vi "auto.vi"() -> ()   [LabVIEW 2010, in "LASA Beta.lvrbt"]
uses:
  LASA Beta.lvrbt
  <vilib>/NXT/Block Support/NXT_ButtonSelector.ctl
  <vilib>/NXT/Dual Mode Library/Display/clearDisplay.vi
  <vilib>/NXT/Dual Mode Library/Display/drawText.vi
  <vilib>/NXT/Dual Mode Library/Sensors/readNXTButton.vi
  <vilib>/NXT/Dual Mode Library/Waits/Wait_Num(msec).vi
  <vilib>/NXT/Dual Mode Library/Display/drawNumber.vi
  op-init.vi
  op-run.vi
  op-read.vi
panel:
  out "IR Success":bool
  in  "Distance":dbl=5750.0
  out "Enabled":bool
  out "Team Number":string="4290"
  in  "Other":dbl
  in  "Ramp":dbl
  in  "Direction":dbl
  in  "Time Delay":dbl
  in  "Cursor":dbl
  # "INITIALIZATION"
  # "Set this number to display team information"
  # "AUTONOMOUS"
  # "If enabled, use robot is on as read by comm. loop"
  # "Data from current IR sensor"
  # "Controller state as read by the comm. loop"
  # "Distance Needed to Travel from Start to B1\nEncoder Counts (1/4th degrees)"
  # "Turns ON when IR is detected"
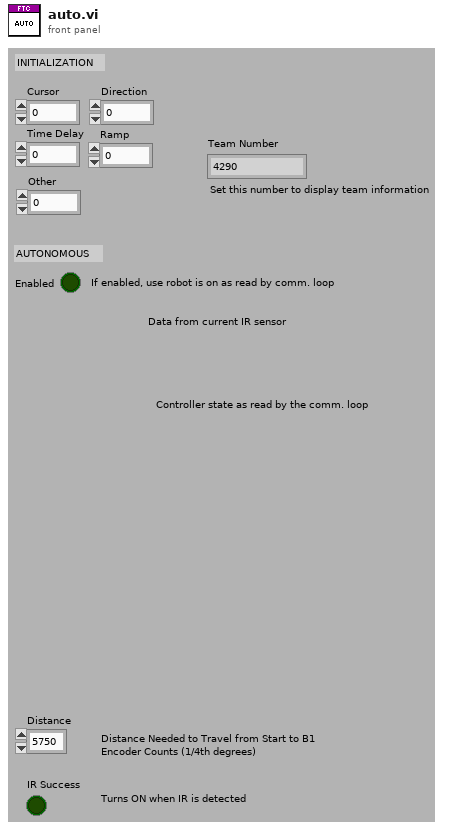
[diagram p1: front panel]
types:
  T1 = typedef "NXT_ButtonSelector.ctl" = u16
  T2 = typedef "LVHSConnector.ctl" = cluster{"Hardware":string, "Flattened String":string}
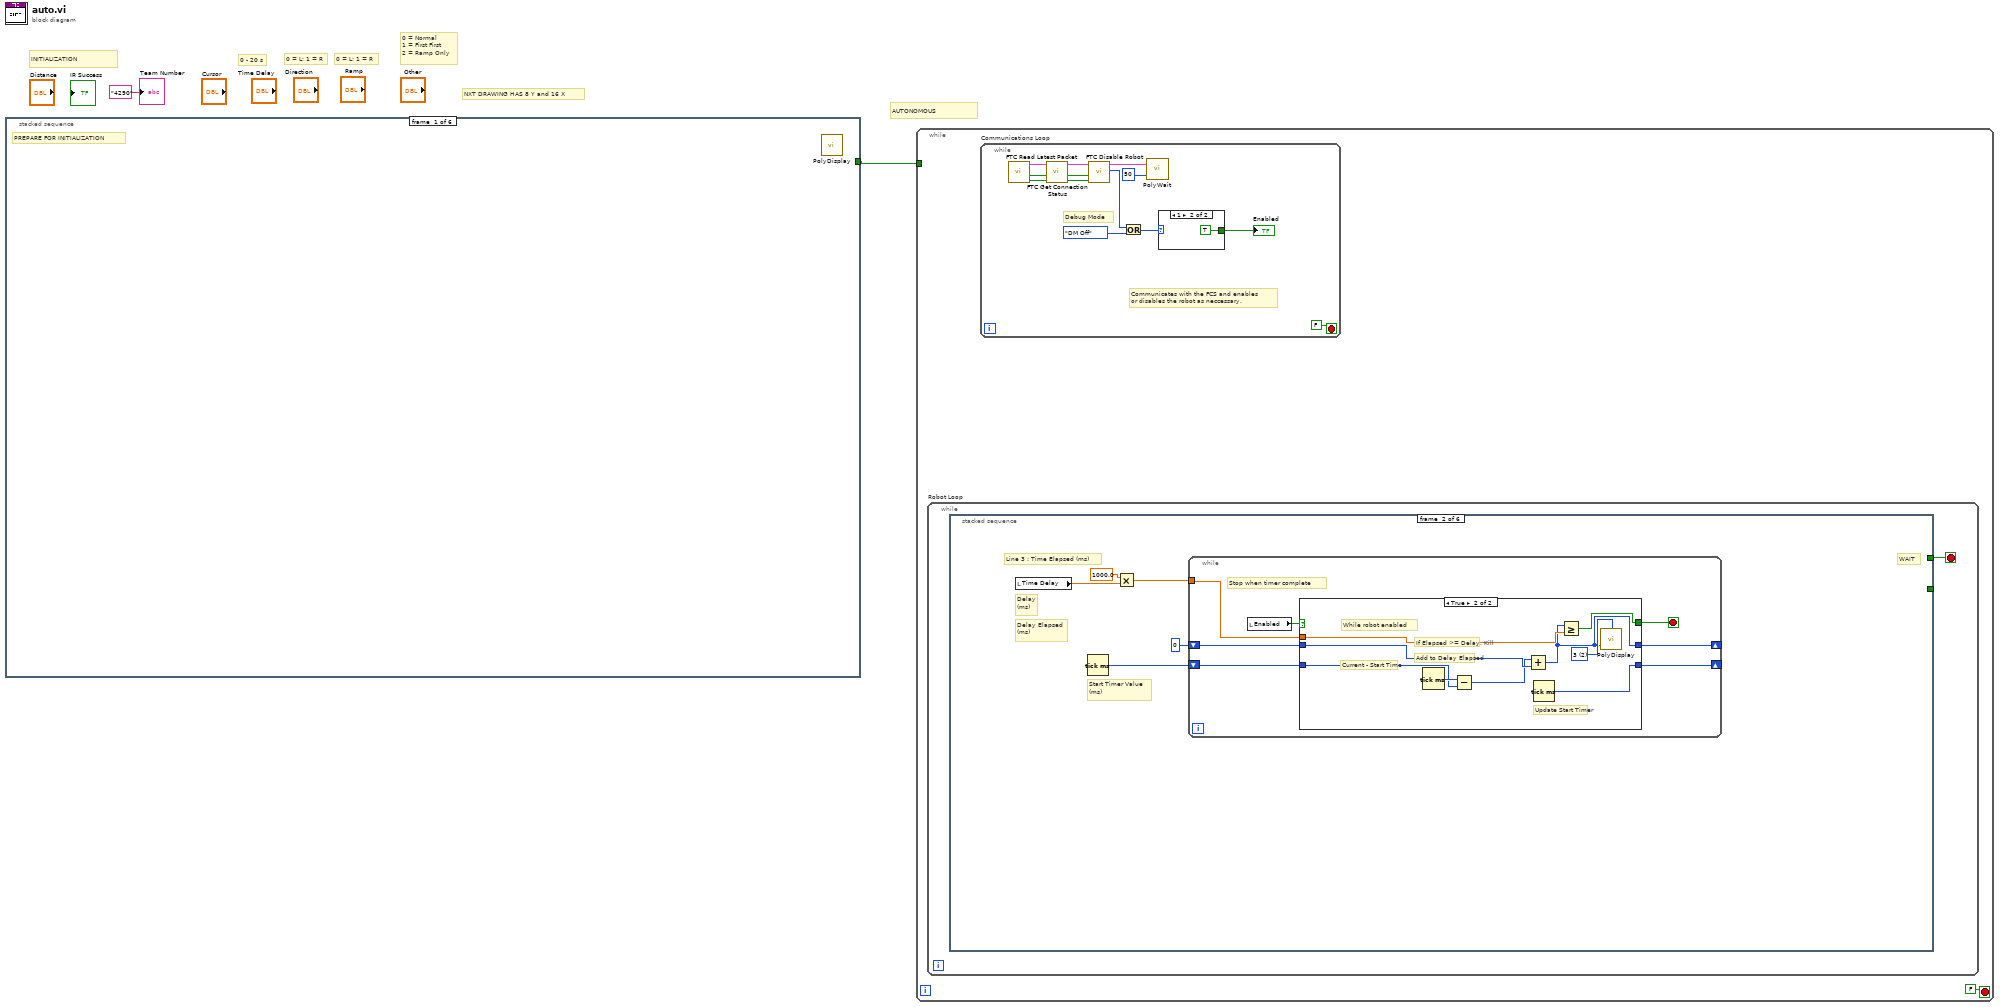
[diagram p0: block diagram]
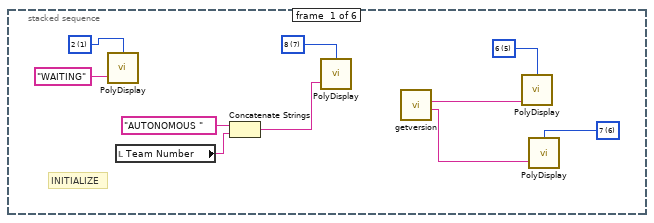
[diagram p2: hidden frame]
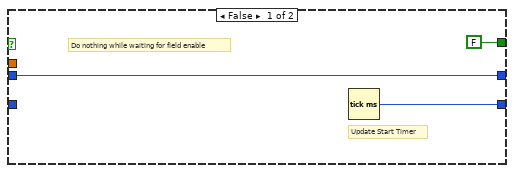
[diagram p3: hidden frame]
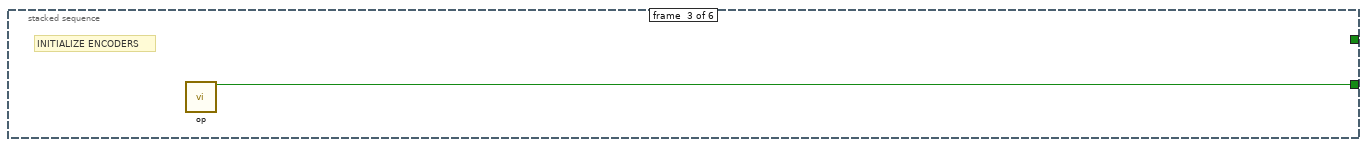
[diagram p4: hidden frame]
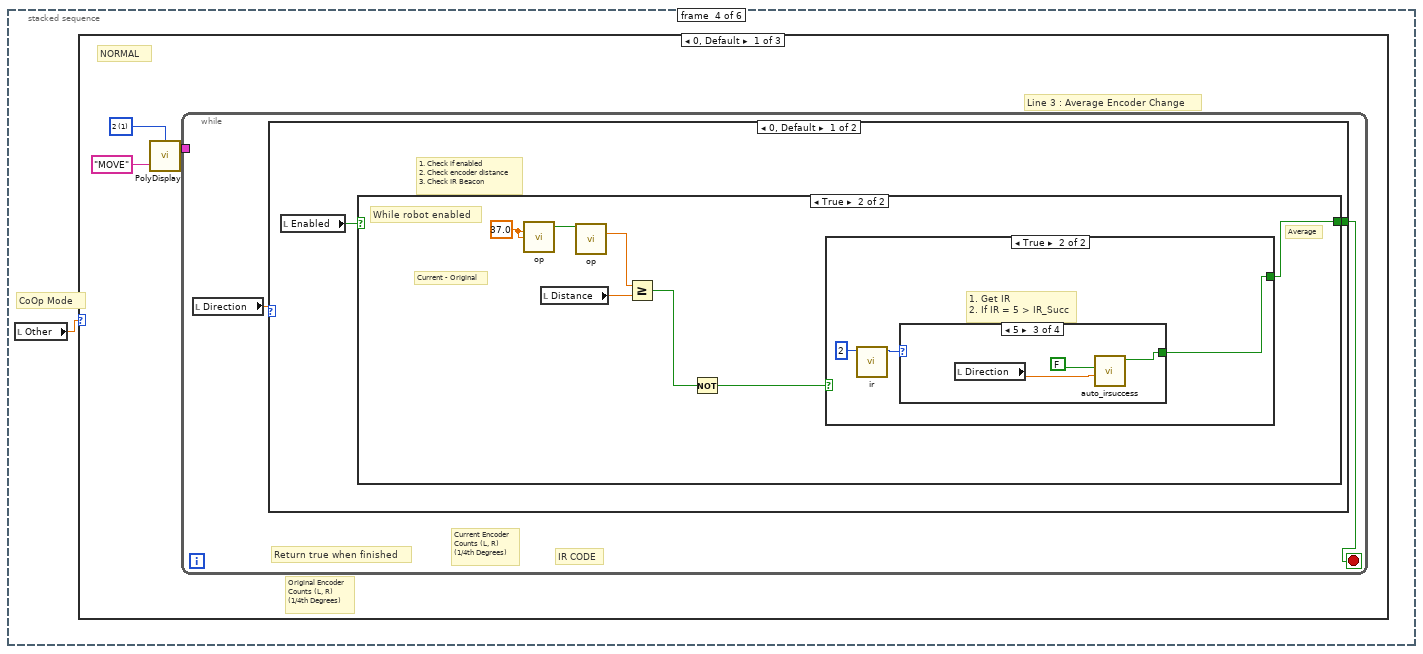
[diagram p5: hidden frame]
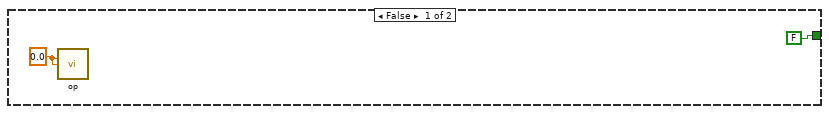
[diagram p6: hidden frame]
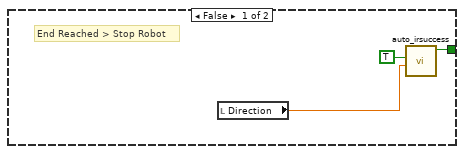
[diagram p7: hidden frame]
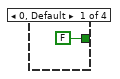
[diagram p8: hidden frame]
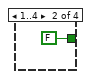
[diagram p9: hidden frame]
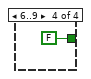
[diagram p10: hidden frame]
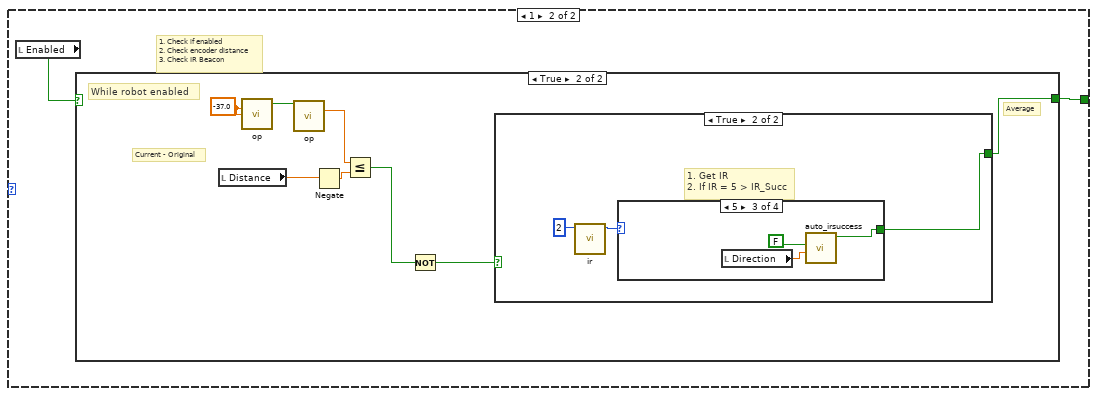
[diagram p11: hidden frame]
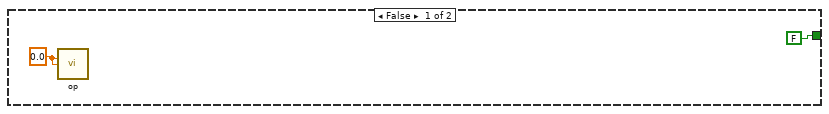
[diagram p12: hidden frame]
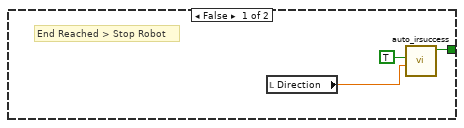
[diagram p13: hidden frame]
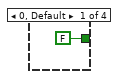
[diagram p14: hidden frame]
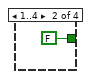
[diagram p15: hidden frame]
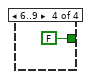
[diagram p16: hidden frame]
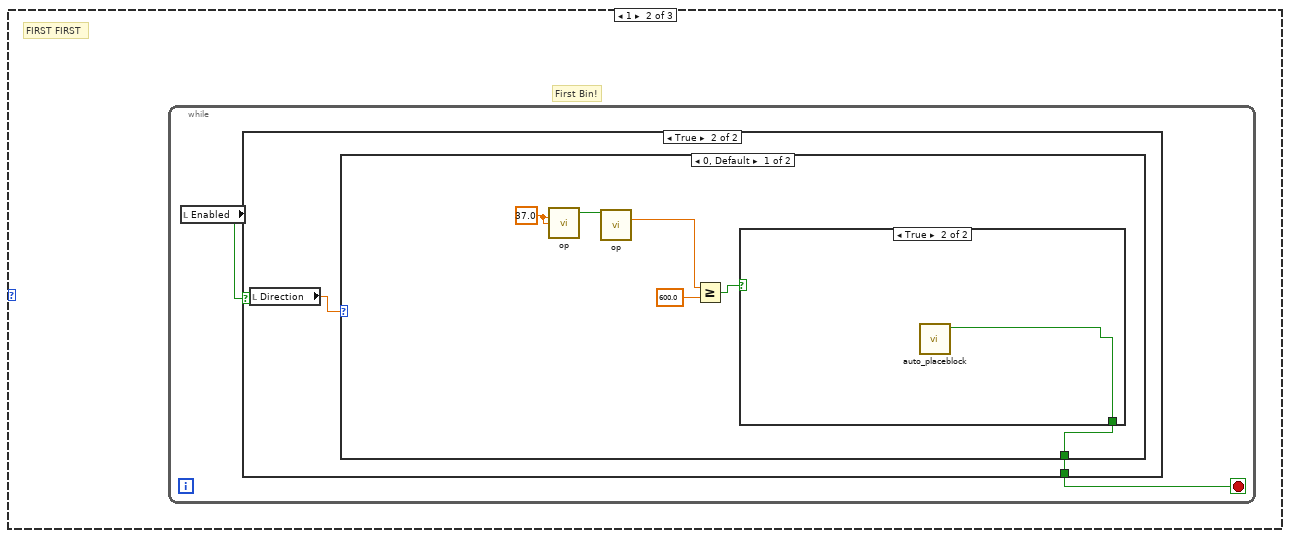
[diagram p17: hidden frame]
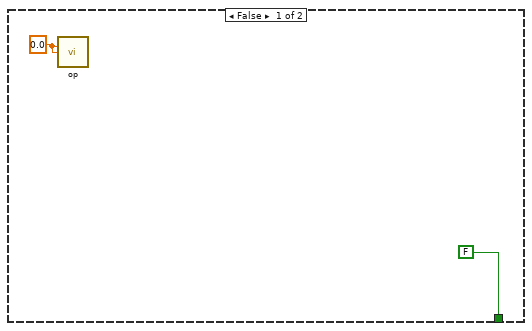
[diagram p18: hidden frame]
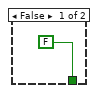
[diagram p19: hidden frame]
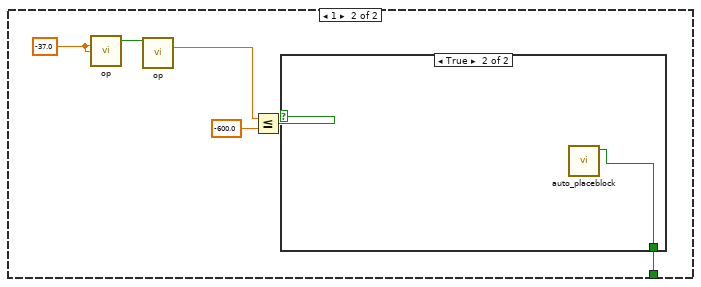
[diagram p20: hidden frame]
diagram:
  # "0 = Normal\n1 = First First\n2 = Ramp Only"
  # "AUTONOMOUS"
  # "INITIALIZATION"
  # "NXT DRAWING HAS 8 Y and 16 X"
  # "0 = L; 1 = R"
  # "0 - 20 s"
  # "0 = L; 1 = R"
  n1 = stacked-sequence {
    tunnel: [_ _ _ _ _ w144] -> w1
    frame #0 {
      # "PREPARE FOR INITIALIZATION"
      n2 = call-poly <vilib>:"PolyDisplay.vi"() -> ()  [unwired: 4 in, 1 out]
    }
    frame #1 {
      n3 = stacked-sequence {
        frame #0 {
          w3 = i16 7 items=["1", "2", "3", "4", "5", "6", "7", "8"] ("Line")
          w11 = i16 2 items=["1", "2", "3", "4", "5", "6", "7", "8"] ("Line")
          w9 = i16 0 items=["1", "2", "3", "4", "5", "6", "7", "8"] ("Line")
          # "-_0 sec_+"
          n4 = local write "Cursor"(0.0 ("Cursor")) -> ()
          n5 = call-poly <vilib>:"PolyDisplay.vi"("Text"="- 0 sec +", "Line"=w11) -> ()  [unwired: 2 in, 1 out]
          n6 = local read "Team Number"() -> (w5:string)
          n7 = call-poly <vilib>:"PolyDisplay.vi"("Text"="TIME DELAY", "Line"=w9) -> ()  [unwired: 2 in, 1 out]
          n8 = Concatenate Strings("AUTONOMOUS " ("string"), w5) -> (w6:string)
          n9 = call-poly <vilib>:"PolyDisplay.vi"("Text"=w6, "Line"=w3) -> ()  [unwired: 2 in, 1 out]
        }
        frame #1 {
          n10 = while {
            stop <- w16 stop-if-true
            w13 = T1 1 items=["Enter button"=3, "Left button"=2, "Right button"=1] ("Button (Enter button)")
            w15 = T1 2 items=["Enter button"=3, "Left button"=2, "Right button"=1] ("Button (Enter button)")
            w18 = T1 3 items=["Enter button"=3, "Left button"=2, "Right button"=1] ("Button (Enter button)")
            n11 = call-poly <vilib>:"PolySensor.vi"("Button (Enter button)"=w15) -> ("Yes/No"=w14:bool)  [unwired: 2 in, 1 out]
            n12 = call-poly <vilib>:"PolySensor.vi"("Button (Enter button)"=w13) -> ("Yes/No"=w12:bool)  [unwired: 2 in, 1 out]
            n13 = call-poly <vilib>:"PolySensor.vi"("Button (Enter button)"=w18) -> ("Yes/No"=w17:bool)  [unwired: 2 in, 1 out]
            n14 = case shown="True" w14 {
              frame False {
              }
              frame True {
                n15 = local read "Cursor"() -> (w41:dbl)
                n16 = Greater?(x=w41, y=0.0) -> (0:w40:bool)
                n17 = case shown="True" w40 {
                  frame False {
                  }
                  frame True {
                    w45 = i16 2 items=["1", "2", "3", "4", "5", "6", "7", "8"] ("Line")
                    n18 = local read "Cursor"() -> (w50:dbl)
                    n19 = Wait (ms)(milliseconds to wait=u32 300) -> ()  [unwired: 1 out]
                    n20 = Subtract(x=w50, y=5.0) -> (x-y=w49:dbl)
                    n21 = local write "Cursor"(w49) -> ()
                    n22 = call <vilib>:"NXT_floatToString.vi"("number"=w49) -> ("string"=w46:string)
                    n23 = Concatenate Strings("- " ("string"), w46, " sec +" ("string")) -> (w44:string)
                    n24 = call-poly <vilib>:"PolyDisplay.vi"("Text"=w44, "Line"=w45) -> ()  [unwired: 2 in, 1 out]
                  }
                }
              }
            }
            n25 = case shown="True" w12 {
              frame False {
              }
              frame True {
                n26 = local read "Cursor"() -> (w21:dbl)
                n27 = Less?(x=w21, y=20.0) -> (x < y?=w19:bool)
                n28 = case shown="True" w19 {
                  frame False {
                  }
                  frame True {
                    w25 = i16 2 items=["1", "2", "3", "4", "5", "6", "7", "8"] ("Line")
                    n29 = local read "Cursor"() -> (w29:dbl)
                    n30 = Wait (ms)(milliseconds to wait=u32 300) -> ()  [unwired: 1 out]
                    n31 = Add(x=w29, y=5.0) -> (x+y=w23:dbl)
                    n32 = local write "Cursor"(w23) -> ()
                    n33 = call <vilib>:"NXT_floatToString.vi"("number"=w23) -> ("string"=w27:string)
                    n34 = Concatenate Strings("- " ("string"), w27, " sec +" ("string")) -> (w26:string)
                    n35 = call-poly <vilib>:"PolyDisplay.vi"("Text"=w26, "Line"=w25) -> ()  [unwired: 2 in, 1 out]
                  }
                }
              }
            }
            n36 = case shown="True" w17 {
              tunnel: [FALSE w32] -> w16
              frame False {
              }
              frame True {
                n37 = stacked-sequence {
                  tunnel: [_ _ TRUE] -> w32
                  frame #0 {
                    n38 = local read "Cursor"() -> (w34:dbl)
                    n39 = local write "Direction"(0.0 ("Direction")) -> ()
                    n40 = local write "Time Delay"(w34) -> ()
                    n41 = call-poly <vilib>:"PolyDisplay.vi"() -> ()  [unwired: 4 in, 1 out]
                  }
                  frame #1 {
                    w37 = i16 0 items=["1", "2", "3", "4", "5", "6", "7", "8"] ("Line")
                    n42 = local write "Cursor"(0.0 ("Cursor")) -> ()
                    n43 = call-poly <vilib>:"PolyDisplay.vi"("Text"="Working...", "Line"=w37) -> ()  [unwired: 2 in, 1 out]
                  }
                  frame #2 {
                    n44 = Wait (ms)(milliseconds to wait=u32 500) -> ()  [unwired: 1 out]
                  }
                }
              }
            }
          }
        }
      }
    }
    frame #2 {
      # "2 = L/R"
      n45 = stacked-sequence {
        frame #0 {
          w52 = i16 3 items=["1", "2", "3", "4", "5", "6", "7", "8"] ("Line")
          w57 = i16 7 items=["1", "2", "3", "4", "5", "6", "7", "8"] ("Line")
          w61 = i16 2 items=["1", "2", "3", "4", "5", "6", "7", "8"] ("Line")
          w59 = i16 0 items=["1", "2", "3", "4", "5", "6", "7", "8"] ("Line")
          n46 = local read "Team Number"() -> (w54:string)
          n47 = call-poly <vilib>:"PolyDisplay.vi"("Text"="[LEFT] = L", "Line"=w61) -> ()  [unwired: 2 in, 1 out]
          n48 = call-poly <vilib>:"PolyDisplay.vi"("Text"="[RIGHT] = R", "Line"=w52) -> ()  [unwired: 2 in, 1 out]
          n49 = Concatenate Strings("AUTONOMOUS " ("string"), w54) -> (w53:string)
          n50 = call-poly <vilib>:"PolyDisplay.vi"("Text"="START LOCATION", "Line"=w59) -> ()  [unwired: 2 in, 1 out]
          n51 = call-poly <vilib>:"PolyDisplay.vi"("Text"=w53, "Line"=w57) -> ()  [unwired: 2 in, 1 out]
        }
        frame #1 {
          n52 = while {
            stop <- w62 stop-if-true
            w67 = T1 1 items=["Enter button"=3, "Left button"=2, "Right button"=1] ("Button (Enter button)")
            w68 = T1 2 items=["Enter button"=3, "Left button"=2, "Right button"=1] ("Button (Enter button)")
            n53 = call-poly <vilib>:"PolySensor.vi"("Button (Enter button)"=w68) -> ("Yes/No"=w65:bool)  [unwired: 2 in, 1 out]
            n54 = call-poly <vilib>:"PolySensor.vi"("Button (Enter button)"=w67) -> ("Yes/No"=w66:bool)  [unwired: 2 in, 1 out]
            n55 = case shown="True" w65 {
              tunnel: [FALSE TRUE] -> w64
              frame False {
              }
              frame True {
                n56 = local write "Direction"(0.0 ("Direction")) -> ()
              }
            }
            n57 = case shown="True" w66 {
              tunnel: [FALSE TRUE] -> w63
              frame False {
              }
              frame True {
                n58 = local write "Direction"(1.0 ("Direction")) -> ()
              }
            }
            n59 = Or(x=w64, y=w63) -> (x .or. y?=w62:bool)
          }
        }
        frame #2 {
          n60 = local write "Cursor"(0.0 ("Cursor")) -> ()
          n61 = local write "Ramp"(0.0 ("Ramp")) -> ()
          n62 = call-poly <vilib>:"PolyDisplay.vi"() -> ()  [unwired: 4 in, 1 out]
        }
        frame #3 {
          w78 = i16 0 items=["1", "2", "3", "4", "5", "6", "7", "8"] ("Line")
          n63 = call-poly <vilib>:"PolyDisplay.vi"("Text"="Working...", "Line"=w78) -> ()  [unwired: 2 in, 1 out]
        }
        frame #4 {
          n64 = Wait (ms)(milliseconds to wait=u32 500) -> ()  [unwired: 1 out]
        }
      }
    }
    frame #3 {
      # "3 = Force On Ramp (L/R)"
      n65 = stacked-sequence {
        frame #0 {
          w81 = i16 3 items=["1", "2", "3", "4", "5", "6", "7", "8"] ("Line")
          w85 = i16 7 items=["1", "2", "3", "4", "5", "6", "7", "8"] ("Line")
          w89 = i16 2 items=["1", "2", "3", "4", "5", "6", "7", "8"] ("Line")
          w87 = i16 0 items=["1", "2", "3", "4", "5", "6", "7", "8"] ("Line")
          n66 = local read "Team Number"() -> (w80:string)
          n67 = call-poly <vilib>:"PolyDisplay.vi"("Text"="[RIGHT] = R", "Line"=w81) -> ()  [unwired: 2 in, 1 out]
          n68 = call-poly <vilib>:"PolyDisplay.vi"("Text"="FORCE RAMP", "Line"=w87) -> ()  [unwired: 2 in, 1 out]
          n69 = call-poly <vilib>:"PolyDisplay.vi"("Text"="[LEFT] = L", "Line"=w89) -> ()  [unwired: 2 in, 1 out]
          n70 = Concatenate Strings("AUTONOMOUS " ("string"), w80) -> (w82:string)
          n71 = call-poly <vilib>:"PolyDisplay.vi"("Text"=w82, "Line"=w85) -> ()  [unwired: 2 in, 1 out]
        }
        frame #1 {
          n72 = while {
            stop <- w90 stop-if-true
            w95 = T1 1 items=["Enter button"=3, "Left button"=2, "Right button"=1] ("Button (Enter button)")
            w96 = T1 2 items=["Enter button"=3, "Left button"=2, "Right button"=1] ("Button (Enter button)")
            n73 = call-poly <vilib>:"PolySensor.vi"("Button (Enter button)"=w96) -> ("Yes/No"=w94:bool)  [unwired: 2 in, 1 out]
            n74 = call-poly <vilib>:"PolySensor.vi"("Button (Enter button)"=w95) -> ("Yes/No"=w93:bool)  [unwired: 2 in, 1 out]
            n75 = case shown="True" w94 {
              tunnel: [FALSE TRUE] -> w92
              frame False {
              }
              frame True {
                n76 = local write "Ramp"(0.0 ("Ramp")) -> ()
              }
            }
            n77 = case shown="True" w93 {
              tunnel: [FALSE TRUE] -> w91
              frame False {
              }
              frame True {
                n78 = local write "Ramp"(1.0 ("Ramp")) -> ()
              }
            }
            n79 = Or(x=w92, y=w91) -> (x .or. y?=w90:bool)
          }
        }
        frame #2 {
          n80 = local write "Cursor"(0.0 ("Cursor")) -> ()
          n81 = local write "Other"(0.0 ("Other")) -> ()
          n82 = call-poly <vilib>:"PolyDisplay.vi"() -> ()  [unwired: 4 in, 1 out]
        }
        frame #3 {
          w106 = i16 0 items=["1", "2", "3", "4", "5", "6", "7", "8"] ("Line")
          n83 = call-poly <vilib>:"PolyDisplay.vi"("Text"="Working...", "Line"=w106) -> ()  [unwired: 2 in, 1 out]
        }
        frame #4 {
          n84 = Wait (ms)(milliseconds to wait=u32 500) -> ()  [unwired: 1 out]
        }
      }
    }
    frame #4 {
      # "4 = Ramp Only, First Bin, or Normal"
      n85 = stacked-sequence {
        frame #0 {
          w108 = i16 4 items=["1", "2", "3", "4", "5", "6", "7", "8"] ("Line")
          w111 = i16 3 items=["1", "2", "3", "4", "5", "6", "7", "8"] ("Line")
          w115 = i16 7 items=["1", "2", "3", "4", "5", "6", "7", "8"] ("Line")
          w119 = i16 2 items=["1", "2", "3", "4", "5", "6", "7", "8"] ("Line")
          w117 = i16 0 items=["1", "2", "3", "4", "5", "6", "7", "8"] ("Line")
          n86 = local read "Team Number"() -> (w110:string)
          n87 = call-poly <vilib>:"PolyDisplay.vi"("Text"="[L] = First Bin", "Line"=w111) -> ()  [unwired: 2 in, 1 out]
          n88 = Concatenate Strings("AUTONOMOUS " ("string"), w110) -> (w112:string)
          n89 = call-poly <vilib>:"PolyDisplay.vi"("Text"="[R] = Ramp Only", "Line"=w108) -> ()  [unwired: 2 in, 1 out]
          n90 = call-poly <vilib>:"PolyDisplay.vi"("Text"="COOPERATION MODE", "Line"=w117) -> ()  [unwired: 2 in, 1 out]
          n91 = call-poly <vilib>:"PolyDisplay.vi"("Text"="[ENTER] = Normal", "Line"=w119) -> ()  [unwired: 2 in, 1 out]
          n92 = call-poly <vilib>:"PolyDisplay.vi"("Text"=w112, "Line"=w115) -> ()  [unwired: 2 in, 1 out]
        }
        frame #1 {
          n93 = while {
            stop <- w124 stop-if-true
            w128 = T1 3 items=["Enter button"=3, "Left button"=2, "Right button"=1] ("Button (Enter button)")
            w129 = T1 1 items=["Enter button"=3, "Left button"=2, "Right button"=1] ("Button (Enter button)")
            w130 = T1 2 items=["Enter button"=3, "Left button"=2, "Right button"=1] ("Button (Enter button)")
            n94 = call-poly <vilib>:"PolySensor.vi"("Button (Enter button)"=w130) -> ("Yes/No"=w127:bool)  [unwired: 2 in, 1 out]
            n95 = call-poly <vilib>:"PolySensor.vi"("Button (Enter button)"=w129) -> ("Yes/No"=w126:bool)  [unwired: 2 in, 1 out]
            n96 = case shown="True" w127 {
              tunnel: [FALSE TRUE] -> w121
              frame False {
              }
              frame True {
                n97 = local write "Other"(1.0 ("Other")) -> ()
              }
            }
            n98 = case shown="True" w126 {
              tunnel: [FALSE TRUE] -> w120
              frame False {
              }
              frame True {
                n99 = local write "Other"(2.0 ("Other")) -> ()
              }
            }
            n100 = call-poly <vilib>:"PolySensor.vi"("Button (Enter button)"=w128) -> ("Yes/No"=w125:bool)  [unwired: 2 in, 1 out]
            n101 = case shown="True" w125 {
              tunnel: [FALSE TRUE] -> w122
              frame False {
              }
              frame True {
                n102 = local write "Other"(0.0 ("Other")) -> ()
              }
            }
            n103 = Or(x=w121, y=w120) -> (x .or. y?=w123:bool)
            n104 = Or(x=w123, y=w122) -> (x .or. y?=w124:bool)
          }
        }
        frame #2 {
          n105 = local write "Cursor"(0.0 ("Cursor")) -> ()
          n106 = call-poly <vilib>:"PolyDisplay.vi"() -> ()  [unwired: 4 in, 1 out]
        }
        frame #3 {
          w142 = i16 0 items=["1", "2", "3", "4", "5", "6", "7", "8"] ("Line")
          n107 = call-poly <vilib>:"PolyDisplay.vi"("Text"="Working...", "Line"=w142) -> ()  [unwired: 2 in, 1 out]
        }
        frame #4 {
          n108 = Wait (ms)(milliseconds to wait=u32 500) -> ()  [unwired: 1 out]
        }
      }
    }
    frame #5 {
      # "ENTER AUTONOMOUS"
      n109 = stacked-sequence {
        tunnel: [_ _ FALSE] -> w144
        frame #0 {
          n110 = call-poly <vilib>:"PolyDisplay.vi"() -> ()  [unwired: 4 in, 1 out]
        }
        frame #1 {
          w148 = i16 7 items=["1", "2", "3", "4", "5", "6", "7", "8"] ("Line")
          n111 = local read "Team Number"() -> (w145:string)
          n112 = Concatenate Strings("AUTONOMOUS " ("string"), w145) -> (w146:string)
          n113 = call-poly <vilib>:"PolyDisplay.vi"("Text"=w146, "Line"=w148) -> ()  [unwired: 2 in, 1 out]
        }
        frame #2 {
        }
      }
    }
  }
  n114 = while {
    tunnel: w1 -> [_]
    stop <- FALSE stop-if-true
    n115 = while "Robot Loop" {
      stop <- w151 stop-if-true
      n116 = stacked-sequence {
        tunnel: [_ _ _ _ _ TRUE] -> w151
        tunnel: [_ _ w186 _ _ _] -> _
        frame #0 {
          w152 = i16 5 items=["1", "2", "3", "4", "5", "6", "7", "8"] ("Line")
          w153 = i16 6 items=["1", "2", "3", "4", "5", "6", "7", "8"] ("Line")
          w159 = i16 7 items=["1", "2", "3", "4", "5", "6", "7", "8"] ("Line")
          w161 = i16 1 items=["1", "2", "3", "4", "5", "6", "7", "8"] ("Line")
          # "INITIALIZE"
          n117 = call-poly <vilib>:"PolyDisplay.vi"("Text"="WAITING", "Line"=w161) -> ()  [unwired: 2 in, 1 out]
          n118 = local read "Team Number"() -> (w157:string)
          n119 = Concatenate Strings("AUTONOMOUS " ("string"), w157) -> (w156:string)
          n120 = call-poly <vilib>:"PolyDisplay.vi"("Text"=w156, "Line"=w159) -> ()  [unwired: 2 in, 1 out]
          n121 = call "getversion.vi"() -> ("Revision"=w154:string, "Version"=w155:string)  [unwired: 9 in, 1 out]
          n122 = call-poly <vilib>:"PolyDisplay.vi"("Text"=w155, "Line"=w152) -> ()  [unwired: 2 in, 1 out]
          n123 = call-poly <vilib>:"PolyDisplay.vi"("Text"=w154, "Line"=w153) -> ()  [unwired: 2 in, 1 out]
        }
        frame #1 {
          # "Line 3 : Time Elapsed (ms)"
          # "Delay\n(ms)"
          # "Start Timer Value\n(ms)"
          # "Delay Elapsed\n(ms)"
          # "WAIT"
          n124 = local read "Time Delay"() -> (w165:dbl)
          n125 = Tick Count (ms)() -> (millisecond timer value=w162:u32)
          n126 = Multiply(x=1000.0, y=w165) -> (x*y=w163:dbl)
          n127 = while {
            shift-right: [w167] -> _
            shift-left: 0 -> [w170]
            tunnel: w163 -> [w172]
            shift-right: [w169] -> _
            shift-left: w162 -> [w171]
            stop <- w168 stop-if-true
            # "Stop when timer complete"
            n128 = local read "Enabled"() -> (w173:bool)
            n129 = case shown="True" w173 {
              tunnel: w172 -> [_ w181]
              tunnel: w171 -> [_ w182]
              tunnel: w170 -> [w175 w184]
              tunnel: [w176 w179] -> w169
              tunnel: [FALSE w180] -> w168
              tunnel: [w175 w177] -> w167
              frame False {
                # "Do nothing while waiting for field enable"
                # "Update Start Timer"
                n130 = Tick Count (ms)() -> (millisecond timer value=w176:u32)
              }
              frame True {
                w178 = i16 2 items=["1", "2", "3", "4", "5", "6", "7", "8"] ("Line")
                # "Update Start Timer"
                # "If Elapsed >= Delay, Kill"
                # "Add to Delay Elapsed"
                # "Current - Start Time"
                # "While robot enabled"
                n131 = Tick Count (ms)() -> (millisecond timer value=w185:u32)
                n132 = Subtract(x=w185, y=w182) -> (x-y=w183:u32)
                n133 = Add(x=w183, y=w184) -> (x+y=w177:u32)
                n134 = Tick Count (ms)() -> (millisecond timer value=w179:u32)
                n135 = Greater Or Equal?(x=w177, y=w181) -> (x >= y?=w180:bool)
                n136 = call-poly <vilib>:"PolyDisplay.vi"("number"=w177, "Line"=w178) -> ()  [unwired: 2 in, 1 out]
              }
            }
          }
        }
        frame #2 {
          # "INITIALIZE ENCODERS"
          n137 = call-poly "op.vi"() -> ("Chain OUT"=w186:bool)  [unwired: 15 in]
        }
        frame #3 {
          # "CoOp Mode"
          n138 = local read "Other"() -> (w187:dbl)
          n139 = case shown="0, Default" w187 {
            frame 0, Default {
              w190 = i16 1 items=["1", "2", "3", "4", "5", "6", "7", "8"] ("Line")
              # "NORMAL"
              # "Line 3 : Average Encoder Change"
              # "Original Encoder\nCounts (L, R)\n(1/4th Degrees)"
              n140 = call-poly <vilib>:"PolyDisplay.vi"("Text"="MOVE", "Line"=w190) -> ("NXT"=w188:T2)  [unwired: 2 in]
              n141 = while {
                tunnel: w188 -> [_]
                stop <- w192 stop-if-true
                # "IR CODE"
                # "Current Encoder\nCounts (L, R)\n(1/4th Degrees)"
                # "Return true when finished"
                n142 = local read "Direction"() -> (w191:dbl)
                n143 = case shown="0, Default" w191 {
                  tunnel: [w193 w216] -> w192
                  frame 0, Default {
                    # "1. Check if enabled\n2. Check encoder distance\n3. Check IR Beacon"
                    n144 = local read "Enabled"() -> (w194:bool)
                    n145 = case shown="True" w194 {
                      tunnel: [FALSE w199] -> w193
                      frame False {
                        w195 = 0.0 ("Left Drive")
                        n146 = call-poly "op.vi"("Left Drive"=w195, "Right Drive"=w195) -> ()  [unwired: 13 in, 1 out]
                      }
                      frame True {
                        w203 = 37.0
                        # "Average"
                        # "Current - Original"
                        # "While robot enabled"
                        n147 = call-poly "op.vi"("Left Drive"=w203, "Right Drive"=w203) -> ("Chain OUT"=w198:bool)  [unwired: 13 in]
                        n148 = local read "Distance"() -> (w202:dbl)
                        n149 = call-poly "op.vi"("Chain IN"=w198) -> ("Encoder Left Drive"=w197:dbl)  [unwired: 8 in, 6 out]
                        n150 = Greater Or Equal?(x=w197, y=w202) -> (x >= y?=w201:bool)
                        n151 = Not(x=w201) -> (.not. x?=w200:bool)
                        n152 = case shown="True" w200 {
                          tunnel: [w205 w209] -> w199
                          frame False {
                            # "End Reached > Stop Robot"
                            n153 = local read "Direction"() -> (w204:dbl)
                            n154 = call "auto_irsuccess.vi"("Direction"=w204, "Skip IR"=TRUE) -> ("Success"=w205:bool)  [unwired: 9 in]
                          }
                          frame True {
                            # "1. Get IR\n2. If IR = 5 > IR_Succ"
                            n155 = call "ir.vi"("Port"=u8 2) -> ("Direction"=w208:i16)  [unwired: 10 in]
                            n156 = case shown="5" w208 {
                              tunnel: [FALSE ("Success") FALSE w214 FALSE] -> w209
                              frame 0, Default {
                              }
                              frame 1..4 {
                              }
                              frame 5 {
                                n157 = local read "Direction"() -> (w212:dbl)
                                n158 = call "auto_irsuccess.vi"("Direction"=w212, "Skip IR"=FALSE) -> ("Success"=w214:bool)  [unwired: 9 in]
                              }
                              frame 6..9 {
                              }
                            }
                          }
                        }
                      }
                    }
                  }
                  frame 1 {
                    # "1. Check if enabled\n2. Check encoder distance\n3. Check IR Beacon"
                    n159 = local read "Enabled"() -> (w217:bool)
                    n160 = case shown="True" w217 {
                      tunnel: [FALSE w223] -> w216
                      frame False {
                        w218 = 0.0 ("Left Drive")
                        n161 = call-poly "op.vi"("Left Drive"=w218, "Right Drive"=w218) -> ()  [unwired: 13 in, 1 out]
                      }
                      frame True {
                        w227 = -37.0
                        # "Average"
                        # "Current - Original"
                        # "While robot enabled"
                        n162 = local read "Distance"() -> (w226:dbl)
                        n163 = call-poly "op.vi"("Left Drive"=w227, "Right Drive"=w227) -> ("Chain OUT"=w222:bool)  [unwired: 13 in]
                        n164 = call-poly "op.vi"("Chain IN"=w222) -> ("Encoder Left Drive"=w221:dbl)  [unwired: 8 in, 6 out]
                        n165 = Negate(x=w226) -> (-x=w220:dbl)
                        n166 = Less Or Equal?(x=w221, y=w220) -> (x <= y?=w225:bool)
                        n167 = Not(x=w225) -> (.not. x?=w224:bool)
                        n168 = case shown="True" w224 {
                          tunnel: [w229 w233] -> w223
                          frame False {
                            # "End Reached > Stop Robot"
                            n169 = local read "Direction"() -> (w228:dbl)
                            n170 = call "auto_irsuccess.vi"("Direction"=w228, "Skip IR"=TRUE) -> ("Success"=w229:bool)  [unwired: 9 in]
                          }
                          frame True {
                            # "1. Get IR\n2. If IR = 5 > IR_Succ"
                            n171 = call "ir.vi"("Port"=u8 2) -> ("Direction"=w232:i16)  [unwired: 10 in]
                            n172 = case shown="5" w232 {
                              tunnel: [FALSE ("Success") FALSE w238 FALSE] -> w233
                              frame 0, Default {
                              }
                              frame 1..4 {
                              }
                              frame 5 {
                                n173 = local read "Direction"() -> (w236:dbl)
                                n174 = call "auto_irsuccess.vi"("Direction"=w236, "Skip IR"=FALSE) -> ("Success"=w238:bool)  [unwired: 9 in]
                              }
                              frame 6..9 {
                              }
                            }
                          }
                        }
                      }
                    }
                  }
                }
              }
            }
            frame 1 {
              # "FIRST FIRST"
              # "First Bin!"
              n175 = while {
                stop <- w241 stop-if-true
                n176 = local read "Enabled"() -> (w240:bool)
                n177 = case shown="True" w240 {
                  tunnel: [FALSE w244] -> w241
                  frame False {
                    w243 = 0.0 ("Left Drive")
                    n178 = call-poly "op.vi"("Left Drive"=w243, "Right Drive"=w243) -> ()  [unwired: 13 in, 1 out]
                  }
                  frame True {
                    n179 = local read "Direction"() -> (w245:dbl)
                    n180 = case shown="0, Default" w245 {
                      tunnel: [w246 w254] -> w244
                      frame 0, Default {
                        w251 = 37.0
                        n181 = call-poly "op.vi"("Left Drive"=w251, "Right Drive"=w251) -> ("Chain OUT"=w250:bool)  [unwired: 13 in]
                        n182 = call-poly "op.vi"("Chain IN"=w250) -> ("Encoder Left Drive"=w247:dbl)  [unwired: 8 in, 6 out]
                        n183 = Greater Or Equal?(x=w247, y=600.0) -> (x >= y?=w248:bool)
                        n184 = case shown="True" w248 {
                          tunnel: [FALSE w253] -> w246
                          frame False {
                          }
                          frame True {
                            n185 = call "auto_placeblock.vi"() -> ("Chain OUT"=w253:bool)  [unwired: 11 in]
                          }
                        }
                      }
                      frame 1 {
                        w259 = -37.0
                        n186 = call-poly "op.vi"("Left Drive"=w259, "Right Drive"=w259) -> ("Chain OUT"=w258:bool)  [unwired: 13 in]
                        n187 = call-poly "op.vi"("Chain IN"=w258) -> ("Encoder Left Drive"=w257:dbl)  [unwired: 8 in, 6 out]
                        n188 = Less Or Equal?(x=w257, y=-600.0) -> (x <= y?=w255:bool)
                        n189 = case shown="True" w255 {
                          tunnel: [FALSE w261] -> w254
                          frame False {
                          }
                          frame True {
                            n190 = call "auto_placeblock.vi"() -> ("Chain OUT"=w261:bool)  [unwired: 11 in]
                          }
                        }
                      }
                    }
                  }
                }
              }
            }
            frame 2 {
              # "Ramp Only, Skip"
            }
          }
        }
        frame #4 {
          w264 = i16 1 items=["1", "2", "3", "4", "5", "6", "7", "8"] ("Line")
          # "RAMP CODE"
          n191 = call-poly <vilib>:"PolyDisplay.vi"("Text"="RAMP", "Line"=w264) -> ("NXT"=w262:T2)  [unwired: 2 in]
          n192 = while {
            tunnel: w262 -> [_]
            stop <- w265 stop-if-true
            n193 = local read "Enabled"() -> (w266:bool)
            n194 = case shown="True" w266 {
              tunnel: [FALSE w269] -> w265
              frame False {
                w267 = 0.0 ("Left Drive")
                n195 = call-poly "op.vi"("Left Drive"=w267, "Right Drive"=w267) -> ()  [unwired: 13 in, 1 out]
              }
              frame True {
                # "REPLACE WITH RAMP MOVEMENT BLOCK!"
                n196 = call "auto_rampnav.vi"() -> ("Complete"=w269:bool)  [unwired: 11 in]
              }
            }
          }
        }
        frame #5 {
          w270 = 0.0 ("Left Drive")
          w272 = i16 1 items=["1", "2", "3", "4", "5", "6", "7", "8"] ("Line")
          # "KILL LOOP"
          n197 = call-poly <vilib>:"PolyDisplay.vi"("Text"="COMPLETE!", "Line"=w272) -> ()  [unwired: 2 in, 1 out]
          n198 = call-poly "op.vi"("Left Drive"=w270, "Right Drive"=w270) -> ()  [unwired: 13 in, 1 out]
        }
      }
    }
    n199 = while "Communications Loop" {
      stop <- FALSE stop-if-true
      # "Debug Mode"
      # "Communicates with the FCS and enables \nor disables the robot as neccessary."
      n200 = call <vilib>:"FTC Read Latest Packet.vi"() -> ("Packet Received?"=w284:bool, "Stopped?"=w283:bool, "NXT"=w286:T2)  [unwired: 6 in, 3 out]
      n201 = call <vilib>:"FTC Get Connection Status.vi"("Packet Received?"=w284, "Stopped?"=w283, "NXT"=w286) -> ("Online?"=w278:bool, "Stopped?"=w279:bool, "NXT"=w285:T2)  [unwired: 5 in]
      n202 = call <vilib>:"FTC Disable Robot.vi"("Online?"=w278, "Stopped?"=w279, "NXT"=w285) -> ("Enabled?"=w276:enum16{"Disabled", "Enabled"}, "NXT"=w281:T2)  [unwired: 3 in]
      n203 = Or(x=w276, y=enum16{"DM Off", "DM On"}."DM Off") -> (x .or. y?=w275:u16)
      n204 = call-poly <vilib>:"PolyWait.vi"("Time (100 msec)"=u32 50 ("Time (msec)"), "NXT"=w281) -> ()  [unwired: 2 in, 1 out]
      n205 = case shown="1" w275 {
        tunnel: [FALSE TRUE] -> w274
        frame 0, Default {
        }
        frame 1 {
        }
      }
      "Enabled" <- w274
    }
  }
  "Team Number" <- "4290" ("Team Number")
